vi "initialize.vi"(8 "error in (no error)":errorcluster, 11 "Hamamatsu_C9100-13 in":refnum<class "Hamamatsu_C9100-13.lvclass">) -> (0 "error out":errorcluster, 3 "Hamamatsu_C9100-13 out":refnum<class "Hamamatsu_C9100-13.lvclass">)   [LabVIEW 2013, in "Hamamatsu_C9100-13.lvclass"]
uses:
  Hamamatsu_C9100-13.lvclass
  <vilib>/vision/Image Controls.llb/IMAQ Image.ctl
  Hamamatsu_C9100-13.lvclass/Hamamatsu_C9100-13.ctl
  Camera.lvclass
  Globals.vi
panel:
  out "trigger source response":string
  out "trigger mode response":string
  out "Image Buffers Array":T1[](array[typedef])
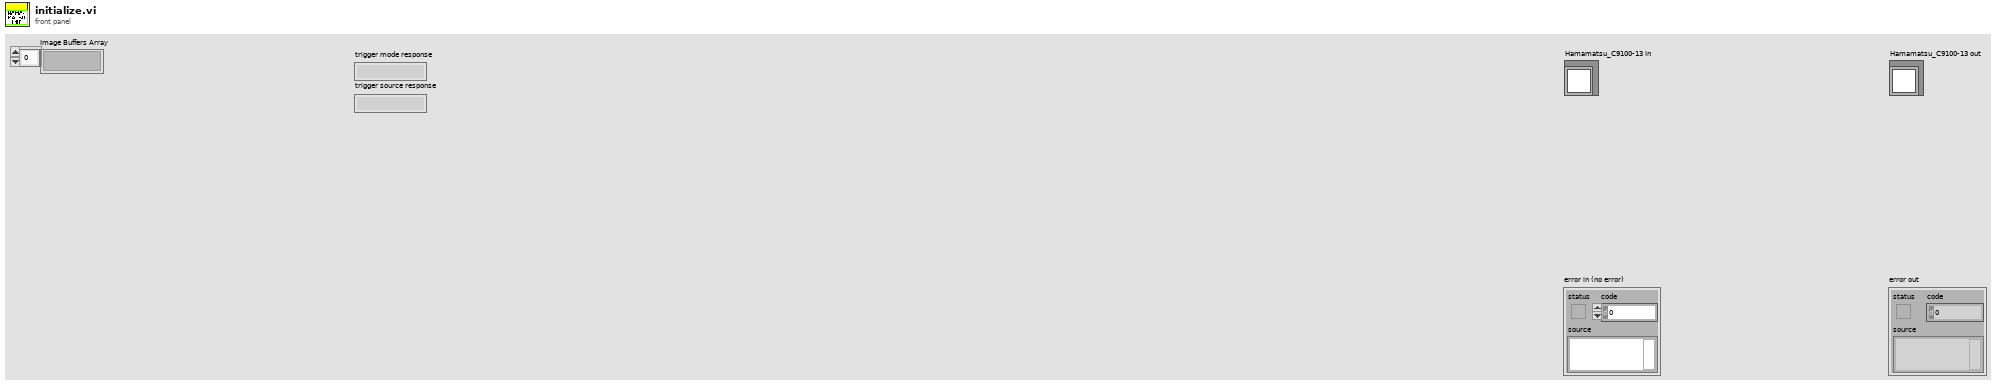
[diagram p1: front panel]
types:
  T1 = typedef "IMAQ Image.ctl" = refnum<image>
  T2 = typedef "Hamamatsu_C9100-13.lvclass/camera_setup.ctl" = cluster{"Analog Gain (0-5)":u8, "Exposure Time":dbl, "EM Gain (0-255)":u8, "Trigger Polarity":string, "External Trigger Mode":string, "Scan Speed":string, "External Trigger Source":string, "Scan Mode":string, "Super Pixel Binning\n(if enabled in Scan Mode)":string, "Camera Sub-array acquisition region\n(if enabled in scan mode)":cluster{"Left":u16, "Top":u16, "Width":u16, "Height":u16}, "Use camera?":bool, "# image buffers":i32, "shots per measurement":i32, "Force images to U16":bool, "Low Light Sensitivity":string, "cooling":string, "fan":string, "Frame Grabber acquisition region":cluster{"Left":i32, "Top":i32, "Right":i32, "Bottom":i32}}
  T3 = cluster{"Left":u16, "Top":u16, "Width":u16, "Height":u16}
  T4 = cluster{"Left":i32, "Top":i32, "Right":i32, "Bottom":i32}
  T5 = typedef "Image Type" = u32
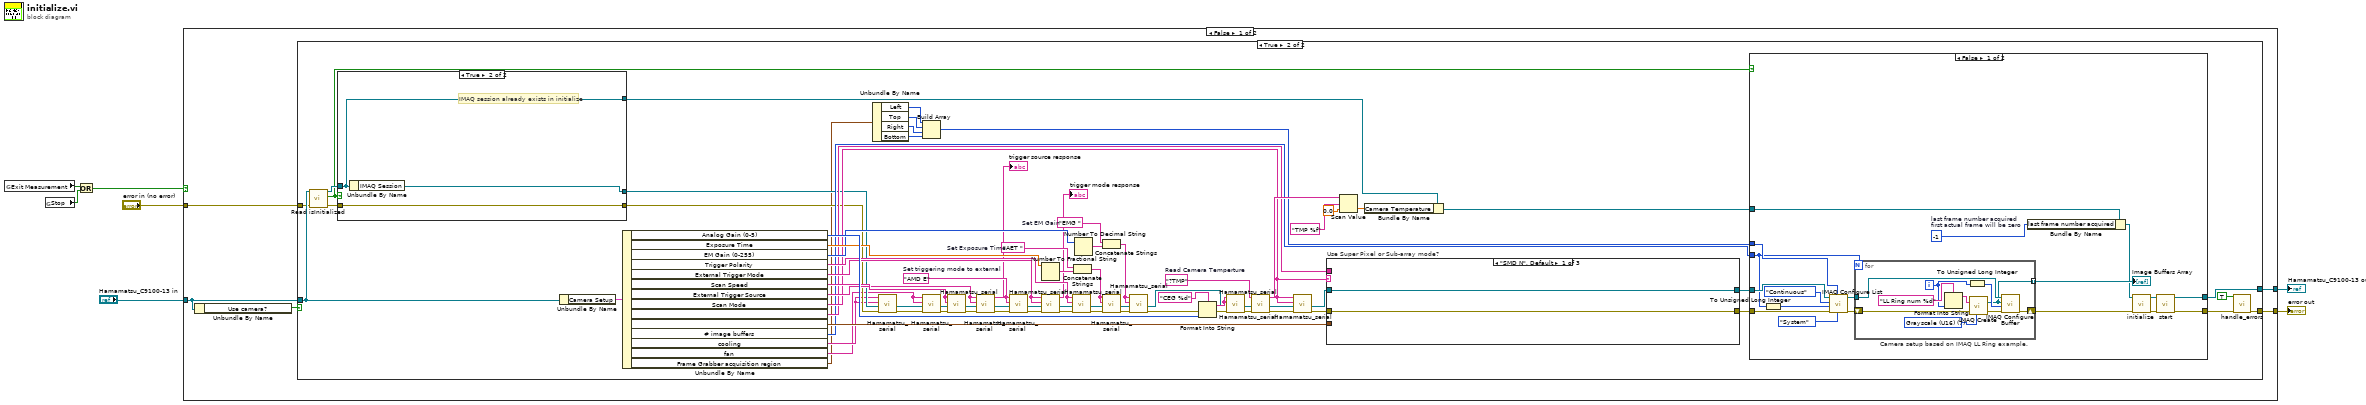
[diagram p0: block diagram]
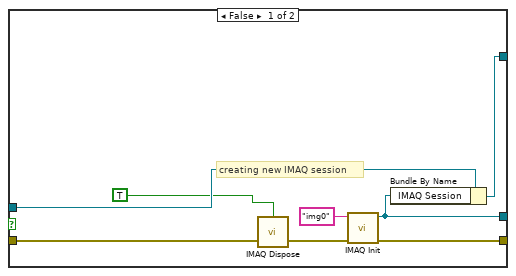
[diagram p4: hidden frame]
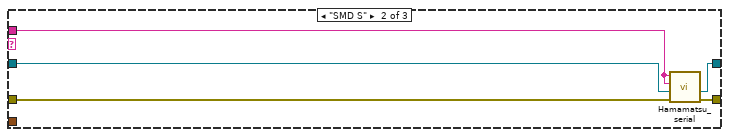
[diagram p5: hidden frame]
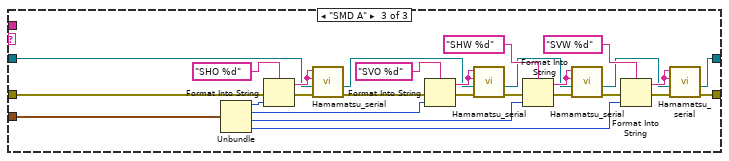
[diagram p6: hidden frame]
diagram:
  n1 = global read "Globals.vi" "Exit Measurement"() -> (w3:bool)
  n2 = global read "Globals.vi" "Stop"() -> (w4:bool)
  n3 = Or(x=w3, y=w4) -> (x .or. y?=w2:bool)
  n4 = case shown="False" w2 {
    tunnel: [w8 w167] -> w7
    tunnel: [w9 w166] -> w6
    tunnel: "Hamamatsu_C9100-13 in" -> [w11 w166]
    tunnel: "error in (no error)" -> [w10 w167]
    frame False {
      n5 = Unbundle By Name(w11) -> ("Use camera?"=w12:bool)
      n6 = case shown="True" w12 {
        tunnel: [w14 w22] -> w8
        tunnel: w10 -> [w14 w17]
        tunnel: w11 -> [w13 w27]
        tunnel: [w13 w16] -> w9
        frame False {
        }
        frame True {
          w87 = "EMG "  # Set EM Gain
          w85 = "AET "  # Set Exposure Time
          w80 = "?TMP"  # Read Camera Temperture
          w90 = "AMD E"  # Set triggering mode to external
          n7 = call-dynamic "Read isInitialized.vi"("error in (no error)"=w17, "Camera in"=w27) -> ("error out"=w51:errorcluster, "isInitialized?"=w19:bool, "Camera out"=w50:refnum<class "Hamamatsu_C9100-13.lvclass">)  [unwired: 7 in]
          n8 = case shown="True" w19 {
            tunnel: [w127 w129] -> w41
            tunnel: w51 -> [w122 w129]
            tunnel: [w124 w131] -> w36
            tunnel: w50 -> [w126 w130]
            tunnel: [w125 w130] -> w18
            frame False {
              # "creating new IMAQ session"
              n9 = call "IMAQ Dispose"("All Images? (No)"=TRUE, "error in (no error)"=w122) -> ("error out"=w121:errorcluster)  [unwired: 4 in]
              n10 = call <vilib>:"IMAQ Init.vi"("error in (no error)"=w121, "Interface Name"="img0") -> ("error out"=w127:errorcluster, "IMAQ Session Out"=w124:refnum<k11>)  [unwired: 8 in]
              n11 = Bundle By Name(cluster=w126, "IMAQ Session"=w124) -> (w125:refnum<class "Hamamatsu_C9100-13.lvclass">)
            }
            frame True {
              # "IMAQ session already exists in initialize"
              n12 = Unbundle By Name(w130) -> ("IMAQ Session"=w131:refnum<k11>)
            }
          }
          n13 = Unbundle By Name(w27) -> ("Camera Setup"=w26:T2)
          n14 = Unbundle By Name(w26) -> ("Analog Gain (0-5)"=w62:u8, "Exposure Time"=w61:dbl, "EM Gain (0-255)"=w60:u8, "Trigger Polarity"=w59:string, "External Trigger Mode"=w58:string, "Scan Speed"=w57:string, "External Trigger Source"=w56:string, "Scan Mode"=w55:string, "Super Pixel Binning\n(if enabled in Scan Mode)"=w54:string, "Camera Sub-array acquisition region\n(if enabled in scan mode)"=w53:T3, "# image buffers"=w52:i32, "cooling"=w35:string, "fan"=w34:string, "Frame Grabber acquisition region"=w33:T4)
          n15 = Unbundle By Name(w33) -> ("Left"=w32:i32, "Top"=w31:i32, "Right"=w30:i32, "Bottom"=w29:i32)
          n16 = call "Hamamatsu_serial.vi"("error in"=w41, "IMAQ Session In"=w36, "Expected Response"=w35, "Command to send"=w35) -> ("error out"=w40:errorcluster, "IMAQ Session Out"=w37:refnum<k11>)  [unwired: 5 in, 1 out]
          n17 = Build Array(w32, w31, w30, w29) -> (w28:i32[])
          n18 = call "Hamamatsu_serial.vi"("error in"=w40, "IMAQ Session In"=w37, "Expected Response"=w34, "Command to send"=w34) -> ("error out"=w39:errorcluster, "IMAQ Session Out"=w38:refnum<k11>)  [unwired: 5 in, 1 out]
          n19 = call "Hamamatsu_serial.vi"("error in"=w39, "IMAQ Session In"=w38, "Expected Response"=w57, "Command to send"=w57) -> ("error out"=w71:errorcluster, "IMAQ Session Out"=w72:refnum<k11>)  [unwired: 5 in, 1 out]
          n20 = call "Hamamatsu_serial.vi"("error in"=w71, "IMAQ Session In"=w72, "Expected Response"=w56, "Command to send"=w56) -> ("error out"=w65:errorcluster, "IMAQ Session Out"=w66:refnum<k11>, "Response from Camera"=→"trigger source response":string)  [unwired: 5 in]
          n21 = call "Hamamatsu_serial.vi"("error in"=w65, "IMAQ Session In"=w66, "Expected Response"=w90, "Command to send"=w90) -> ("error out"=w63:errorcluster, "IMAQ Session Out"=w64:refnum<k11>)  [unwired: 5 in, 1 out]
          n22 = Number To Fractional String(number=w61) -> (F-format string=w86:string)  [unwired: 3 in]
          n23 = call "Hamamatsu_serial.vi"("error in"=w63, "IMAQ Session In"=w64, "Expected Response"=w58, "Command to send"=w58) -> ("error out"=w49:errorcluster, "IMAQ Session Out"=w48:refnum<k11>, "Response from Camera"=→"trigger mode response":string)  [unwired: 5 in]
          n24 = call "Hamamatsu_serial.vi"("error in"=w49, "IMAQ Session In"=w48, "Expected Response"=w59, "Command to send"=w59) -> ("error out"=w74:errorcluster, "IMAQ Session Out"=w73:refnum<k11>)  [unwired: 5 in, 1 out]
          n25 = Concatenate Strings(w85, w86) -> (w84:string)
          n26 = Number To Decimal String(number=w60) -> (decimal integer string=w89:string)  [unwired: 1 in]
          n27 = Concatenate Strings(w87, w89) -> (w88:string)
          n28 = call "Hamamatsu_serial.vi"("error in"=w74, "IMAQ Session In"=w73, "Expected Response"=w84, "Command to send"=w84) -> ("error out"=w46:errorcluster, "IMAQ Session Out"=w47:refnum<k11>)  [unwired: 5 in, 1 out]
          n29 = call "Hamamatsu_serial.vi"("error in"=w46, "IMAQ Session In"=w47, "Expected Response"=w88, "Command to send"=w88) -> ("error out"=w76:errorcluster, "IMAQ Session Out"=w75:refnum<k11>)  [unwired: 5 in, 1 out]
          n30 = Format Into String(format string="CEG %d", error in=w76, w62) -> (resulting string=w78:string, error out=w77:errorcluster)  [unwired: 1 in]
          n31 = call "Hamamatsu_serial.vi"("error in"=w77, "IMAQ Session In"=w75, "Expected Response"=w78, "Command to send"=w78) -> ("error out"=w45:errorcluster, "IMAQ Session Out"=w44:refnum<k11>)  [unwired: 5 in, 1 out]
          n32 = call "Hamamatsu_serial.vi"("error in"=w45, "IMAQ Session In"=w44, "Command to send"=w80) -> ("error out"=w70:errorcluster, "IMAQ Session Out"=w68:refnum<k11>, "Response from Camera"=w82:string)  [unwired: 6 in]
          n33 = call "Hamamatsu_serial.vi"("error in"=w70, "IMAQ Session In"=w68, "Expected Response"=w55, "Command to send"=w55) -> ("error out"=w69:errorcluster, "IMAQ Session Out"=w67:refnum<k11>)  [unwired: 5 in, 1 out]
          n34 = case "Use Super Pixel or Sub-array mode?" shown="\"SMD N\", Default" w55 {
            tunnel: w69 -> [w133 w138 w145]
            tunnel: [w133 w137 w146] -> w43
            tunnel: [w132 w134 w147] -> w42
            tunnel: w67 -> [w132 w135 w144]
            tunnel: w54 -> [_ w136 _]
            tunnel: w53 -> [_ _ w143]
            frame "SMD N", Default {
            }
            frame "SMD S" {
              n35 = call "Hamamatsu_serial.vi"("error in"=w138, "IMAQ Session In"=w135, "Expected Response"=w136, "Command to send"=w136) -> ("error out"=w137:errorcluster, "IMAQ Session Out"=w134:refnum<k11>)  [unwired: 5 in, 1 out]
            }
            frame "SMD A" {
              n36 = Unbundle(w143) -> ("Left"=w142:u16, "Top"=w141:u16, "Width"=w140:u16, "Height"=w139:u16)
              n37 = Format Into String(format string="SHO %d", error in=w145, w142) -> (resulting string=w162:string, error out=w152:errorcluster)  [unwired: 1 in]
              n38 = call "Hamamatsu_serial.vi"("error in"=w152, "IMAQ Session In"=w144, "Expected Response"=w162, "Command to send"=w162) -> ("error out"=w153:errorcluster, "IMAQ Session Out"=w150:refnum<k11>)  [unwired: 5 in, 1 out]
              n39 = Format Into String(format string="SVO %d", error in=w153, w141) -> (resulting string=w163:string, error out=w154:errorcluster)  [unwired: 1 in]
              n40 = call "Hamamatsu_serial.vi"("error in"=w154, "IMAQ Session In"=w150, "Expected Response"=w163, "Command to send"=w163) -> ("error out"=w155:errorcluster, "IMAQ Session Out"=w149:refnum<k11>)  [unwired: 5 in, 1 out]
              n41 = Format Into String(format string="SHW %d", error in=w155, w140) -> (resulting string=w164:string, error out=w156:errorcluster)  [unwired: 1 in]
              n42 = call "Hamamatsu_serial.vi"("error in"=w156, "IMAQ Session In"=w149, "Expected Response"=w164, "Command to send"=w164) -> ("error out"=w157:errorcluster, "IMAQ Session Out"=w148:refnum<k11>)  [unwired: 5 in, 1 out]
              n43 = Format Into String(format string="SVW %d", error in=w157, w139) -> (resulting string=w165:string, error out=w158:errorcluster)  [unwired: 1 in]
              n44 = call "Hamamatsu_serial.vi"("error in"=w158, "IMAQ Session In"=w148, "Expected Response"=w165, "Command to send"=w165) -> ("error out"=w146:errorcluster, "IMAQ Session Out"=w147:refnum<k11>)  [unwired: 5 in, 1 out]
            }
          }
          n45 = Scan Value(string=w82, format string="TMP %f", default (0 dbl)=0.0 ("value (0)")) -> (value=w24:dbl)  [unwired: 1 out]
          n46 = Bundle By Name(cluster=w18, "Camera Temperature"=w24) -> (w25:refnum<class "Hamamatsu_C9100-13.lvclass">)
          n47 = case shown="False" w19 {
            tunnel: w43 -> [w106 w120]
            tunnel: w42 -> [w105 _]
            tunnel: [w93 w120] -> w15
            tunnel: w28 -> [w102 _]
            tunnel: w52 -> [w100 _]
            tunnel: w25 -> [w97 w119]
            tunnel: [w91 w119] -> w16
            frame False {
              w98 = -1  # last frame number acquired first actual frame will be zero
              n48 = To Unsigned Long Integer(number=w100) -> (unsigned 32bit integer=w99:u32)
              n49 = call <vilib>:"IMAQ Configure List.vi"("Memory Location"=enum16{"System", "Onboard"}."System", "Region of interest"=w102, "error in (no error)"=w106, "Number of buffers"=w99, "Continuous?"=enum16{"One-Shot", "Continuous"}."Continuous", "IMAQ Session In"=w105) -> ("error out"=w103:errorcluster, "IMAQ Session Out"=w104:refnum<k11>)  [unwired: 4 in]
              n50 = for "Camera setup based on IMAQ LL Ring example." {
                N: w100 -> [_]
                tunnel: w104 -> [w117]
                shift-right: [w114] -> w95
                shift-left: w103 -> [w118]
                tunnel: [w109] -> w107 mode=indexing
                i -> [w112]
                w113 = T5 7 items=["Grayscale (U8)", "Grayscale (I16)", "Grayscale (SGL)", "Complex (CSG)", "RGB (U32)", "HSL (U32)", "RGB (U64)", "Grayscale (U16)"] ("Image Type")
                n51 = Format Into String(format string="LL Ring num %d", w112) -> (resulting string=w116:string)  [unwired: 2 in, 1 out]
                n52 = To Unsigned Long Integer(number=w112) -> (unsigned 32bit integer=w111:u32)
                n53 = call "IMAQ Create"("Image Name"=w116, "Image Type"=w113, "error in (no error)"=w118) -> ("New Image"=w109:T1, "error out"=w110:errorcluster)  [unwired: 2 in]
                n54 = call <vilib>:"IMAQ Configure Buffer.vi"("error in (no error)"=w110, "Buffer Number"=w111, "Image In"=w109, "IMAQ Session In"=w117) -> ("error out"=w114:errorcluster)  [unwired: 6 in, 1 out]
              }
              "Image Buffers Array" <- w107
              n55 = Bundle By Name(cluster=w97, "last frame number acquired"=w98) -> (w96:refnum<class "Hamamatsu_C9100-13.lvclass">)
              n56 = call-parent "initialize.vi"("error in (no error)"=w95, "Camera in"=w96) -> ("error out"=w94:errorcluster, "Camera out"=w92:refnum<class "Hamamatsu_C9100-13.lvclass">)  [unwired: 8 in]
              n57 = call-dynamic "start.vi"("error in (no error)"=w94, "Hamamatsu_C9100-13 in"=w92) -> ("error out"=w93:errorcluster, "Hamamatsu_C9100-13 out"=w91:refnum<class "Hamamatsu_C9100-13.lvclass">)  [unwired: 8 in]
            }
            frame True {
            }
          }
          n58 = call "handle_errors.vi"("Exit Operation"=TRUE, "error in (no error)"=w15) -> ("error out"=w22:errorcluster)  [unwired: 13 in]
        }
      }
    }
    frame True {
    }
  }
  "error out" <- w7
  "Hamamatsu_C9100-13 out" <- w6
